vi "_SIS_defux_heater.vi"(8 "SIS_Deflux_heater":T1={"ON開始時間（mｓ）"=3000.0, "ON継続時間（mｓ）"=1000.0, "測定終了時間（mｓ）"=60000.0, "SIS Volt（mV)"=0.5, "GPIB_PW (SISHeater) "="3", "SAVE"=TRUE, "file_name"="", "パス"=path "Z:/band10/Labview_ALMA/MIX95/test"}, 11 "Bias_LO_equip":T2={"Node address"=19, "CAN Interface"="CAN0", "Cartridge band"=10, "Slave Node in"={"Address"=19, "Serial Number"=[16, 71, 55, 76, 1, 8, 0, -15]}, "ObjHandle out"=89653312, "POL"=1, "sb"=1, "GPIB_SM (SIS S,V)"="24", "GPIB_DMM (SIS I)"="22", "GPIB_SM (MAG I) "="25", "GPIB_SG(LO)"="19", "GPIB_PW (PAMP) "="6", "GPIB_TMP1(8ch)"="12", "GPIB_TMP2(2ch)  "="13", "WCA_avg"=10, "Rsen"=10.0, "BiasModule"=0, "LOModule "=1, "WCA_LO_FREQ_SET"={"YTO Low freq. [GHz]"=14.42, "YTO High freq. [GHz]"=17.7, "Kvco"=1, "Lock Pol."=0, "SET LO FREQ"=72.5, "Multiplier"=6.0, "YTO (HEX)"=0, "YTO coarse( FREQ)"=25.0, "NULL PLL INTEGRATOR"=FALSE}, "Res for"=0} {"Res for" items=["none", "series res", "parallel res"]; "WCA_LO_FREQ_SET"."YTO coarse( FREQ)" min=25 max=150 step=0.0001 format="%.3f"; "WCA_LO_FREQ_SET"."Multiplier" min=3 max=6 step=3; "WCA_LO_FREQ_SET"."SET LO FREQ" min=25 max=150 step=0.0001 format="%.3f"; "WCA_LO_FREQ_SET"."Lock Pol." items=["Lower", "Upper"]; "WCA_LO_FREQ_SET"."Kvco" items=["7.5MHz/V", "15MHz/V"]; "WCA_LO_FREQ_SET"."YTO High freq. [GHz]" format="%.3f"; "WCA_LO_FREQ_SET"."YTO Low freq. [GHz]" format="%.3f"; "LOModule" items=["Manual", "B10Lab LO", "WCA LO"]; "BiasModule" items=["B10Lab Bias", "WCA BiasModule"]; "Slave Node in"."Serial Number" format="%.0x"; "Slave Node in"."Address" format="%.0x"; "Cartridge band" max=10 step=1; "Node address" format="%.0x"}) -> ()   [LabVIEW 2017]
uses:
  __sub_vi/WCA_NAOJ_sub_vi/WCA_Global.vi
panel:
  out "ON開始（ｍｓ） 2":u32=779747487
  out "Heater":bool
  out "Link済み":bool=TRUE
  out "ON開始（ｍｓ）":u32=779747487
  out "ON終了時間（ｍｓ）":u32=779767487
  out "終了時間（ｍｓ）":u32=779804487
  out "初期時間（ms）":u32=779744487
  out "波形チャート":dbl(graph)
  out "Temp":T3(graph)={"4K_Temp"=3.333, "90/20K_temp"=15.541, "MixTemp"=4.14, "Get_I(uA)"=3.4236999999999997}
  # "LO freq. [GHz]"
  # "YTO LOW\n/High Freq."
  # "ZERO Intgrtr"
  # "Node Address"
  # "Serial Number"
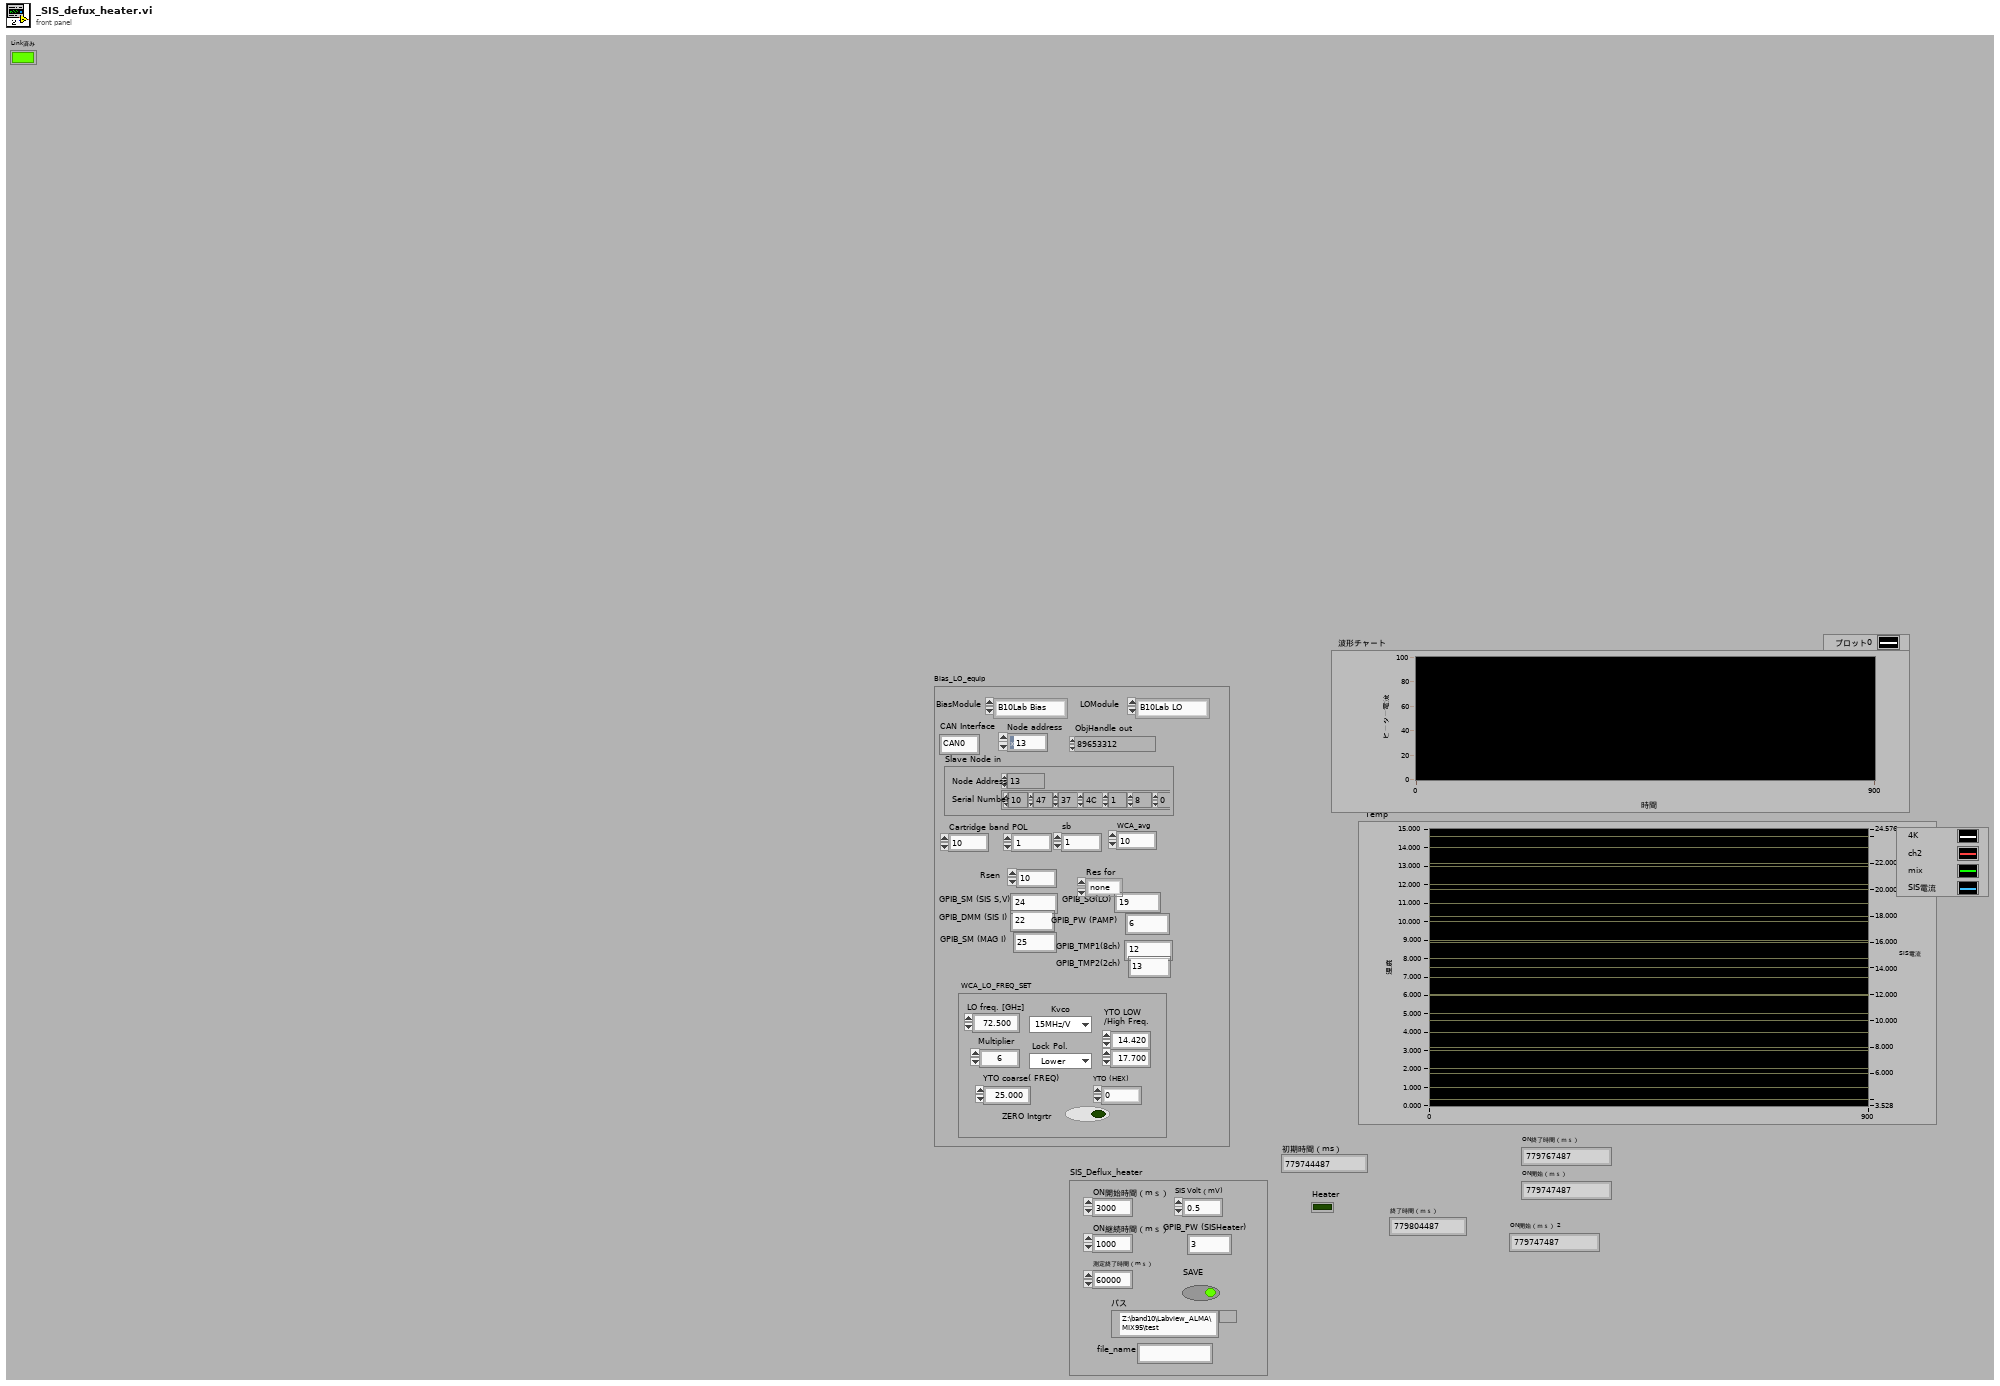
[diagram p1: front panel]
types:
  T1 = cluster{"ON開始時間（mｓ）":dbl, "ON継続時間（mｓ）":dbl, "測定終了時間（mｓ）":dbl, "SIS Volt（mV)":dbl, "GPIB_PW (SISHeater) ":string, "SAVE":bool, "file_name":string, "パス":path}
  T2 = cluster{"Node address":u16, "CAN Interface":string, "Cartridge band":u32, "Slave Node in":cluster{"Address":i16, "Serial Number":i8[]}, "ObjHandle out":u32, "POL":u32, "sb":u32, "GPIB_SM (SIS S,V)":string, "GPIB_DMM (SIS I)":string, "GPIB_SM (MAG I) ":string, "GPIB_SG(LO)":string, "GPIB_PW (PAMP) ":string, "GPIB_TMP1(8ch)":string, "GPIB_TMP2(2ch)  ":string, "WCA_avg":i32, "Rsen":dbl, "BiasModule":u16, "LOModule ":u16, "WCA_LO_FREQ_SET":cluster{"YTO Low freq. [GHz]":sgl, "YTO High freq. [GHz]":sgl, "Kvco":u16, "Lock Pol.":u16, "SET LO FREQ":sgl, "Multiplier":sgl, "YTO (HEX)":u16, "YTO coarse( FREQ)":sgl, "NULL PLL INTEGRATOR":bool}, "Res for":u16}
  T3 = cluster{"4K_Temp":dbl, "90/20K_temp":dbl, "MixTemp":dbl, "Get_I(uA)":dbl}
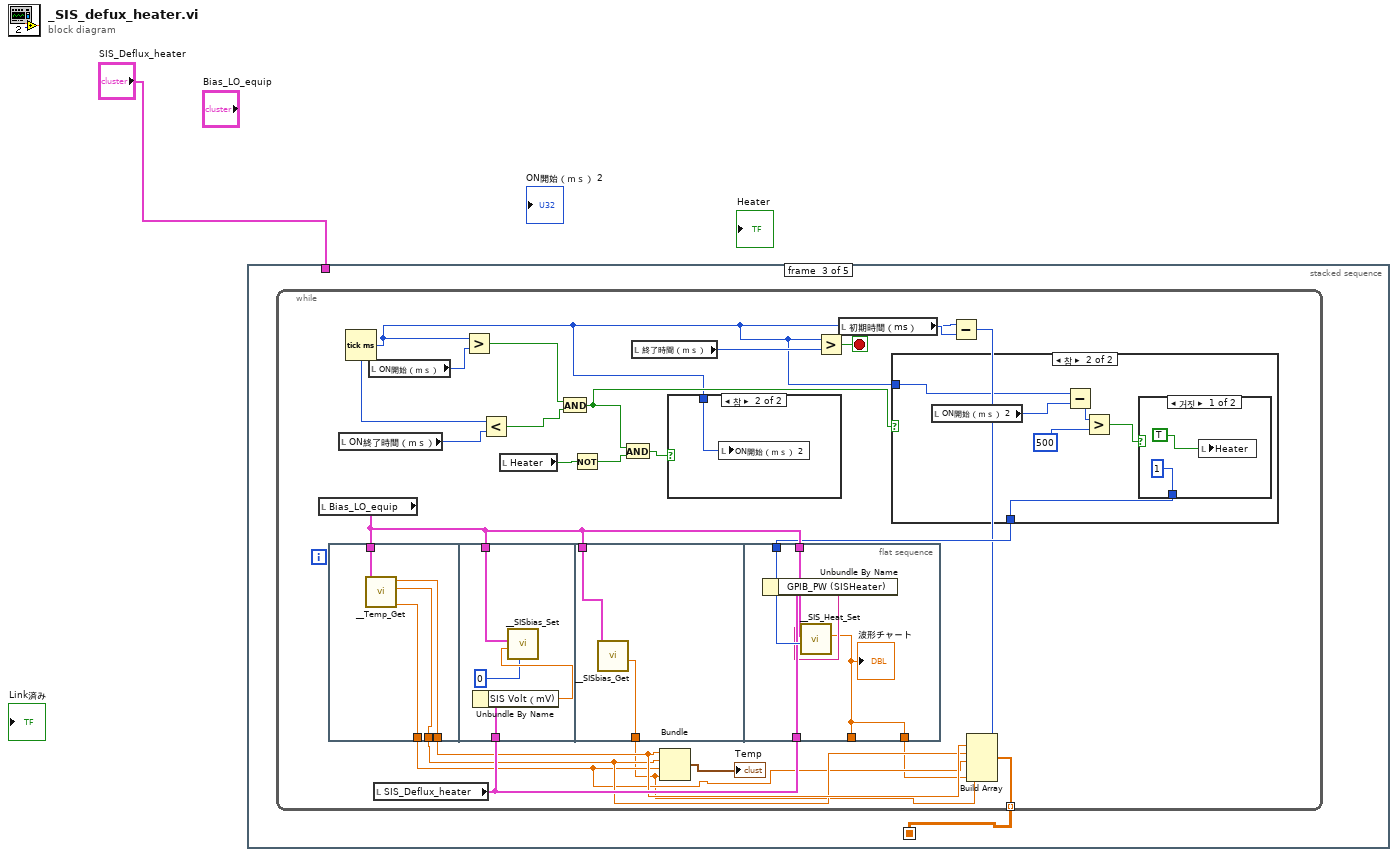
[diagram p0: block diagram]
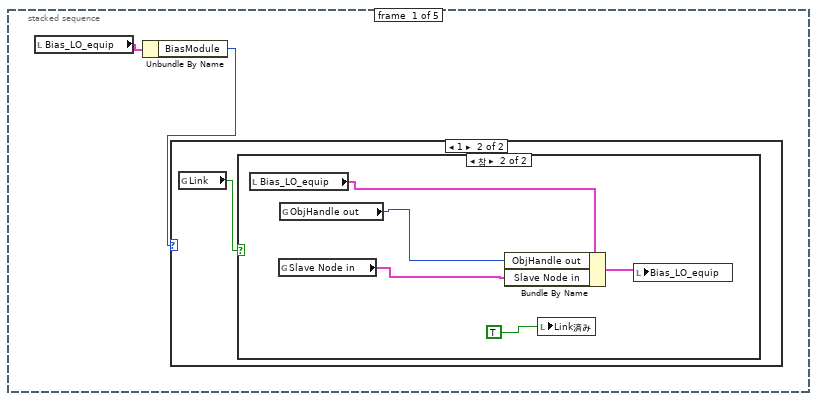
[diagram p2: hidden frame]
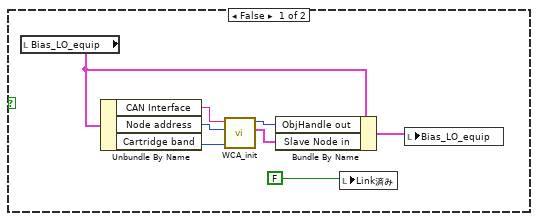
[diagram p4: hidden frame]
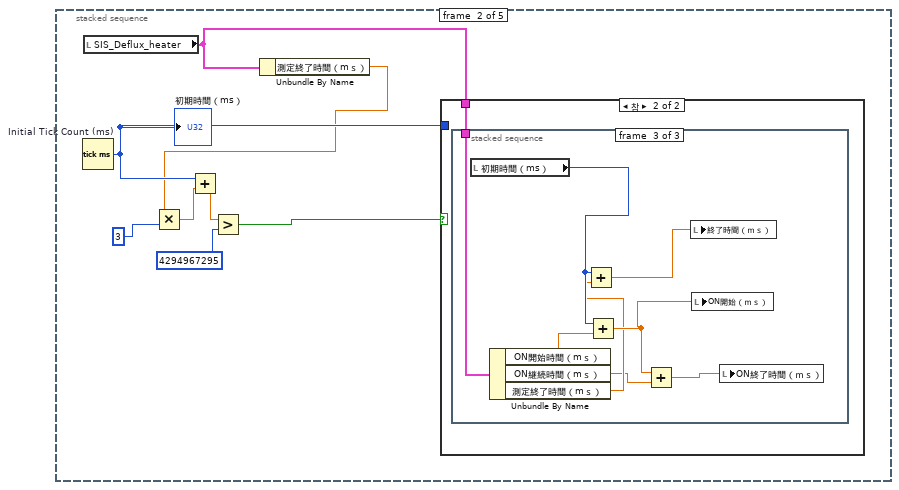
[diagram p5: hidden frame]
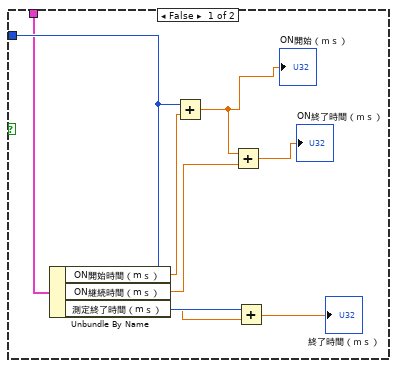
[diagram p6: hidden frame]
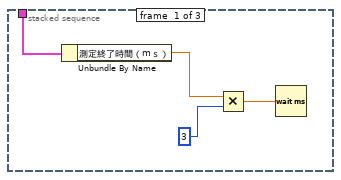
[diagram p7: hidden frame]
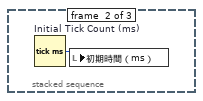
[diagram p8: hidden frame]
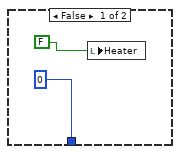
[diagram p10: hidden frame]
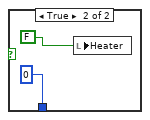
[diagram p11: hidden frame]
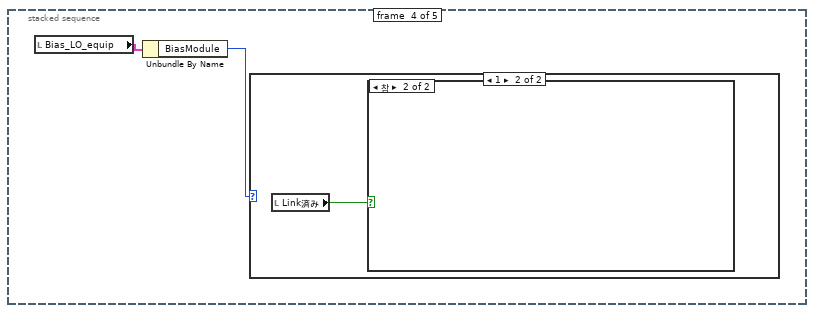
[diagram p12: hidden frame]
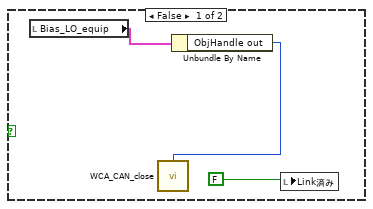
[diagram p14: hidden frame]
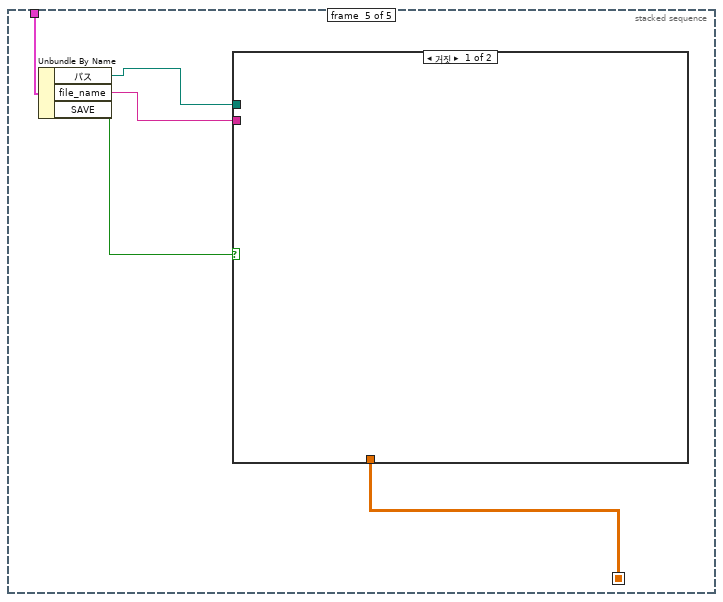
[diagram p15: hidden frame]
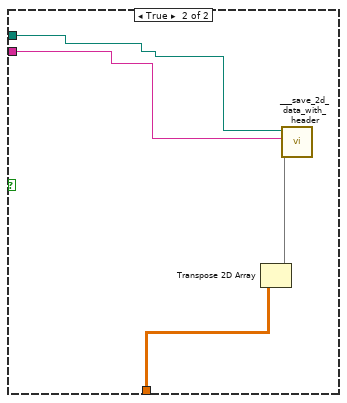
[diagram p16: hidden frame]
diagram:
  n1 = stacked-sequence {
    seq-local: [_ _ w48 _ _] -> [_ _ _ _ w108]
    tunnel: "SIS_Deflux_heater" -> [_ _ _ _ w110]
    frame #0 {
      n2 = local read "Bias_LO_equip"() -> (w3:T2)
      n3 = Unbundle By Name(w3) -> ("BiasModule"=w2:u16)
      n4 = case shown="1" w2 {
        frame 0, Default {
        }
        frame 1 {
          n5 = global read "WCA_Global.vi" "Link"() -> (w4:bool)
          n6 = case shown="참" w4 {
            frame False {
              n7 = local read "Bias_LO_equip"() -> (w5:T2)
              n8 = Unbundle By Name(w5) -> ("CAN Interface"=w9:string, "Node address"=w8:u16, "Cartridge band"=w7:u32)
              n9 = call "WCA_init.vi"("Cartridge band"=w7, "Node address"=w8, "CAN Interface"=w9) -> ("Slave Node in"=w11:cluster{"Address":i16, "Serial Number":i8[]}, "ObjHandle out"=w12:u32)  [unwired: 4 in, 3 out]
              n10 = Bundle By Name(cluster=w5, "ObjHandle out"=w12, "Slave Node in"=w11) -> (w6:T2)
              n11 = local write "Link済み"(FALSE) -> ()
              n12 = local write "Bias_LO_equip"(w6) -> ()
            }
            frame True {
              n13 = local read "Bias_LO_equip"() -> (w16:T2)
              n14 = global read "WCA_Global.vi" "Slave Node in"() -> (w14:cluster{"Address":i16, "Serial Number":i8[]})
              n15 = global read "WCA_Global.vi" "ObjHandle out"() -> (w15:u32)
              n16 = Bundle By Name(cluster=w16, "ObjHandle out"=w15, "Slave Node in"=w14) -> (w17:T2)
              n17 = local write "Link済み"(TRUE) -> ()
              n18 = local write "Bias_LO_equip"(w17) -> ()
            }
          }
        }
      }
    }
    frame #1 {
      n19 = Tick Count (ms) "Initial Tick Count (ms)"() -> (millisecond timer value=w22:u32)
      "初期時間（ms）" <- w22
      n20 = local read "SIS_Deflux_heater"() -> (w18:T1)
      n21 = Unbundle By Name(w18) -> ("測定終了時間（mｓ）"=w20:dbl)
      n22 = Multiply(x=w20, y=3) -> (x*y=w21:dbl)
      n23 = Add(x=w22, y=w21) -> (x+y=w25:dbl)
      n24 = Greater?(x=w25, y=u32 4294967295) -> (0:w23:bool)
      n25 = case shown="참" w23 {
        tunnel: w22 -> [w32 _]
        tunnel: w18 -> [w29 w34]
        frame False {
          n26 = Unbundle By Name(w29) -> ("ON開始時間（mｓ）"=w26:dbl, "ON継続時間（mｓ）"=w27:dbl, "測定終了時間（mｓ）"=w28:dbl)
          n27 = Add(x=w32, y=w26) -> (x+y=w31:dbl)
          "ON開始（ｍｓ）" <- w31
          n28 = Add(x=w31, y=w27) -> (x+y=→"ON終了時間（ｍｓ）":dbl)
          n29 = Add(x=w32, y=w28) -> (x+y=→"終了時間（ｍｓ）":dbl)
        }
        frame True {
          n30 = stacked-sequence {
            tunnel: w34 -> [w35 _ w43]
            frame #0 {
              n31 = Unbundle By Name(w35) -> ("測定終了時間（mｓ）"=w36:dbl)
              n32 = Multiply(x=w36, y=3) -> (x*y=w38:dbl)
              n33 = Wait (ms)(milliseconds to wait=w38) -> ()  [unwired: 1 out]
            }
            frame #1 {
              n34 = Tick Count (ms) "Initial Tick Count (ms)"() -> (millisecond timer value=w39:u32)
              n35 = local write "初期時間（ms）"(w39) -> ()
            }
            frame #2 {
              n36 = local read "初期時間（ms）"() -> (w47:u32)
              n37 = Unbundle By Name(w43) -> ("ON開始時間（mｓ）"=w41:dbl, "ON継続時間（mｓ）"=w40:dbl, "測定終了時間（mｓ）"=w42:dbl)
              n38 = Add(x=w47, y=w42) -> (x+y=w46:dbl)
              n39 = Add(x=w47, y=w41) -> (x+y=w45:dbl)
              n40 = Add(x=w45, y=w40) -> (x+y=w44:dbl)
              n41 = local write "終了時間（ｍｓ）"(w46) -> ()
              n42 = local write "ON開始（ｍｓ）"(w45) -> ()
              n43 = local write "ON終了時間（ｍｓ）"(w44) -> ()
            }
          }
        }
      }
    }
    frame #2 {
      n44 = while {
        tunnel: [w57] -> w48 mode=indexing
        stop <- w67 stop-if-true
        n45 = local read "Bias_LO_equip"() -> (w66:T2)
        n46 = flat-sequence {
          tunnel: w66 -> [w76]
          tunnel: [w75] -> w62
          tunnel: [w74] -> w61
          tunnel: [w73] -> w60
          tunnel: w66 -> [w80]
          tunnel: w64 -> [w79]
          tunnel: w66 -> [w82]
          tunnel: [w81] -> w59
          tunnel: w66 -> [w87]
          tunnel: w65 -> [w86]
          tunnel: w64 -> [w85]
          tunnel: [w83] -> _
          tunnel: [w83] -> w58
          frame #0 {
            n47 = call "__Temp_Get.vi"("Bias_LO_equip"=w76) -> ("MixTemp"=w73:dbl, "90/20K_temp"=w74:dbl, "4K_Temp"=w75:dbl)  [unwired: 8 in]
          }
          frame #1 {
            n48 = Unbundle By Name(w79) -> ("SIS Volt（mV)"=w78:dbl)
            n49 = call "__SISbias_Set.vi"("SIS　Mode"=0, "Set_V"=w78, "Bias_LO_equip"=w80) -> ()  [unwired: 8 in, 1 out]
          }
          frame #2 {
            n50 = call "__SISbias_Get.vi"("Bias_LO_equip"=w82) -> ("Get_I(uA)"=w81:dbl)  [unwired: 8 in, 2 out]
          }
          frame #3 {
            n51 = Unbundle By Name(w85) -> ("GPIB_PW (SISHeater)"=w84:string)
            n52 = call "__SIS_Heat_Set.vi"("Set_Heat_state(0:OFF 1:ON)"=w86, "Bias_LO_equip"=w87, "GPIB_PW (SISHeater)"=w84) -> ("電流"=w83:dbl)  [unwired: 8 in]
            "波形チャート" <- w83
          }
        }
        n53 = local read "ON終了時間（ｍｓ）"() -> (w70:u32)
        n54 = Tick Count (ms)() -> (millisecond timer value=w49:u32)
        n55 = local read "ON開始（ｍｓ）"() -> (w71:u32)
        n56 = local read "SIS_Deflux_heater"() -> (w64:T1)
        n57 = Greater?(x=w49, y=w71) -> (0:w69:bool)
        n58 = Less?(x=w49, y=w70) -> (x < y?=w54:bool)
        n59 = local read "Heater"() -> (w53:bool)
        n60 = And(x=w69, y=w54) -> (x .and. y?=w51:bool)
        n61 = Not(x=w53) -> (.not. x?=w52:bool)
        n62 = And(x=w51, y=w52) -> (x .and. y?=w50:bool)
        n63 = local read "終了時間（ｍｓ）"() -> (w68:u32)
        n64 = Bundle("4K_Temp"=w62, "90/20K_temp"=w61, "MixTemp"=w60, "Get_I(uA)"=w59) -> (→"Temp":T3)  [unwired: 1 in]
        n65 = case shown="참" w50 {
          tunnel: w49 -> [_ w72]
          frame False {
          }
          frame True {
            n66 = local write "ON開始（ｍｓ） 2"(w72) -> ()
          }
        }
        n67 = Greater?(x=w49, y=w68) -> (0:w67:bool)
        n68 = local read "初期時間（ms）"() -> (w55:u32)
        n69 = case shown="참" w51 {
          tunnel: [0 w90] -> w65
          tunnel: w49 -> [_ w95]
          frame False {
            n70 = local write "Heater"(FALSE) -> ()
          }
          frame True {
            n71 = local read "ON開始（ｍｓ） 2"() -> (w94:u32)
            n72 = Subtract(x=w95, y=w94) -> (x-y=w93:u32)
            n73 = Greater?(x=w93, y=500) -> (0:w91:bool)
            n74 = case shown="거짓" w91 {
              tunnel: [1 0] -> w90
              frame False {
                n75 = local write "Heater"(TRUE) -> ()
              }
              frame True {
                n76 = local write "Heater"(FALSE) -> ()
              }
            }
          }
        }
        n77 = Subtract(x=w49, y=w55) -> (x-y=w56:u32)
        n78 = Build Array(w56, w62, w61, w60, w59, w58) -> (w57:dbl[])
      }
    }
    frame #3 {
      n79 = local read "Bias_LO_equip"() -> (w101:T2)
      n80 = Unbundle By Name(w101) -> ("BiasModule"=w100:u16)
      n81 = case shown="1" w100 {
        frame 0, Default {
        }
        frame 1 {
          n82 = local read "Link済み"() -> (w102:bool)
          n83 = case shown="참" w102 {
            frame False {
              n84 = local read "Bias_LO_equip"() -> (w104:T2)
              n85 = Unbundle By Name(w104) -> ("ObjHandle out"=w103:u32)
              n86 = call "WCA_CAN_close.vi"("ObjHandle in"=w103) -> ()  [unwired: 14 in, 1 out]
              n87 = local write "Link済み"(FALSE) -> ()
            }
            frame True {
            }
          }
        }
      }
    }
    frame #4 {
      n88 = Unbundle By Name(w110) -> ("パス"=w107:path, "file_name"=w106:string, "SAVE"=w109:bool)
      n89 = case shown="거짓" w109 {
        tunnel: w108 -> [_ w114]
        tunnel: w107 -> [_ w111]
        tunnel: w106 -> [_ w112]
        frame False {
        }
        frame True {
          n90 = Transpose 2D Array(2D array=w114) -> (transposed array=w113:dbl[][])
          n91 = call "___save_2d_data_with_header.vi"("配列"=w113, "file_name"=w112, "パス"=w111) -> ()  [unwired: 8 in, 1 out]
        }
      }
    }
  }
